vi "ReadDataUV-visSD.vi"(0 "Nombre de aq":i32=2, 1 "Binning Horizontal":i32=1) -> (2 "Channel I":i32[][](array[numeric]), 3 "Channel II":i32[][](array[numeric]), 4 "DLL error code":u32=20066, 5 "temps d'acqu ms":u32=4148)   [LabVIEW 2015]
uses:
  Error Code Enum typedef.ctl
panel:
  out "status":T1=enum."DRV_IDLE"
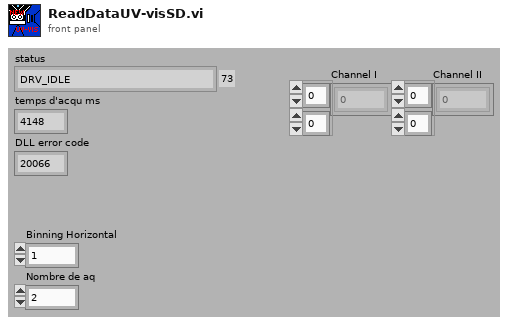
[diagram p1: front panel]
types:
  T1 = typedef "Error Code Enum typedef.ctl" = enum32{"N/A (0)", "DRV_ERROR_CODES", "DRV_SUCCESS", "DRV_VXDNOTINSTALLED", "DRV_ERROR_SCAN", "DRV_ERROR_CHECK_SUM", "DRV_ERROR_FILELOAD", "DRV_UNKNOWN_FUNC", "DRV_ERROR_VXD_INIT", "DRV_ERROR_ADDRESS", "DRV_ERROR_PAGELOCK", "DRV_ERROR_PAGEUNLOCK", "DRV_ERROR_BOARDTEST", "DRV_ERROR_ACK", "DRV_ERROR_UP_FIFO", "DRV_ERROR_PATTERN", "N/A (16)", "DRV_ACQUISITION_ERRORS", "DRV_ACQ_BUFFER", "DRV_ACQ_DOWNFIFO_FULL", "DRV_PROC_UNKONWN_INSTRUCTION", "DRV_ILLEGAL_OP_CODE", "DRV_KINETIC_TIME_NOT_MET", "DRV_ACCUM_TIME_NOT_MET", "DRV_NO_NEW_DATA", "N/A (25)", "DRV_SPOOLERROR", "N/A (27)", "N/A (28)", "N/A (29)", "N/A (30)", "N/A (31)", "N/A (32)", "DRV_TEMPERATURE_CODES", "DRV_TEMPERATURE_OFF", "DRV_TEMPERATURE_NOT_STABILIZED", "DRV_TEMPERATURE_STABILIZED", "DRV_TEMPERATURE_NOT_REACHED", "DRV_TEMPERATURE_OUT_RANGE", "DRV_TEMPERATURE_NOT_SUPPORTED", "DRV_TEMPERATURE_DRIFT", "N/A (41)", "N/A (42)", "N/A (43)", "N/A (44)", "N/A (45)", "N/A (46)", "N/A (47)", "N/A (48)", "DRV_GENERAL_ERRORS", "DRV_INVALID_AUX", "DRV_COF_NOTLOADED", "DRV_FPGAPROG", "DRV_FLEXERROR", "DRV_GPIBERROR", "N/A (55)", "N/A (56)", "N/A (57)", "N/A (58)", "N/A (59)", "N/A (60)", "N/A (61)", "N/A (62)", "N/A (63)", "DRV_DATATYPE", "DRV_DRIVER_ERRORS", "DRV_P1INVALID", "DRV_P2INVALID", "DRV_P3INVALID", "DRV_P4INVALID", "DRV_INIERROR", "DRV_COFERROR", "DRV_ACQUIRING", "DRV_IDLE", "DRV_TEMPCYCLE", "DRV_NOT_INITIALIZED", "DRV_P5INVALID", "DRV_P6INVALID", "DRV_INVALID_MODE", "DRV_INVALID_FILTER", "DRV_I2CERRORS", "DRV_I2CDEVNOTFOUND", "DRV_I2CTIMEOUT", "DRV_P7INVALID", "N/A (84)", "N/A (85)", "N/A (86)", "N/A (87)", "N/A (88)", "N/A (89)", "DRV_IOCERROR", "DRV_VRMVERSIONERROR"}
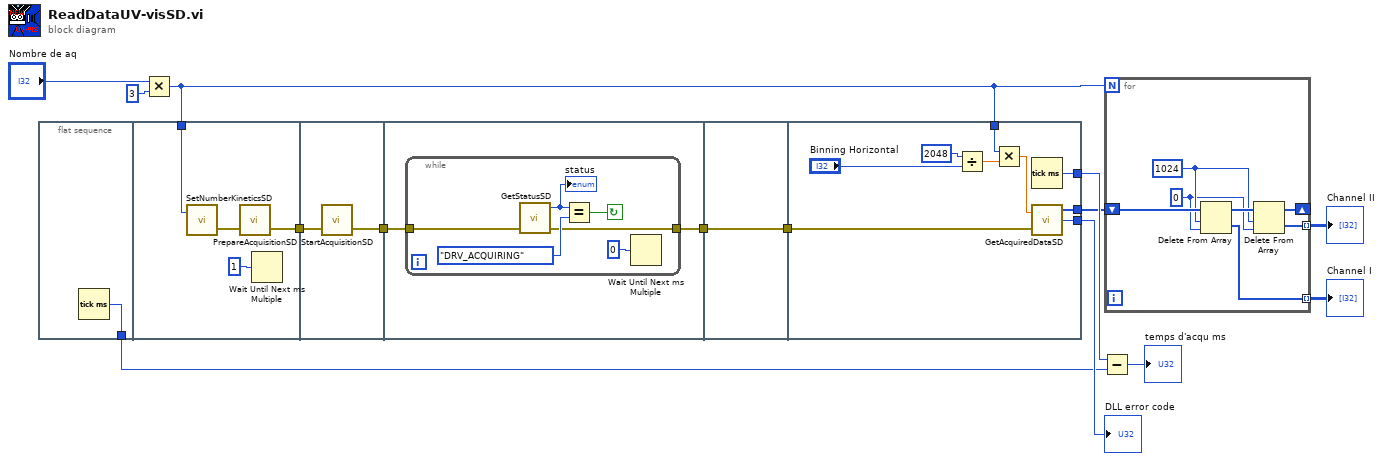
[diagram p0: block diagram]
diagram:
  n1 = flat-sequence {
    tunnel: [w15] -> w8
    tunnel: [w17] -> w12
    tunnel: w4 -> [w16]
    tunnel: w12 -> [w21]
    tunnel: [w20] -> w11
    tunnel: w11 -> [w23]
    tunnel: [w22] -> w9
    tunnel: [w30] -> w10
    tunnel: w9 -> [w30]
    tunnel: [w38] -> w3
    tunnel: [w37] -> w14
    tunnel: w10 -> [w34]
    tunnel: [w33] -> w7
    tunnel: w4 -> [w32]
    frame #0 {
      n2 = Tick Count (ms)() -> (millisecond timer value=w15:u32)
    }
    frame #1 {
      n3 = call "SetNumberKineticsSD.vi"("number"=w16) -> ("error out"=w19:errorcluster)  [unwired: 1 in, 1 out]
      n4 = call "PrepareAcquisitionSD.vi"("error in (no error)"=w19) -> ("error out"=w17:errorcluster)  [unwired: 1 in, 1 out]
      n5 = Wait Until Next ms Multiple(millisecond multiple=u32 1 ("n millisecondes")) -> ()  [unwired: 1 out]
    }
    frame #2 {
      n6 = call "StartAcquisitionSD.vi"("error in (no error)"=w21) -> ("error out"=w20:errorcluster)  [unwired: 1 in, 1 out]
    }
    frame #3 {
      n7 = while {
        tunnel: w23 -> [w25]
        tunnel: [w24] -> w22
        stop <- w27 continue-if-true
        n8 = call "GetStatusSD.vi"("error in (no error)"=w25) -> ("error out"=w24:errorcluster, "status"=w26:T1)  [unwired: 2 in, 1 out]
        "status" <- w26
        n9 = Equal?(x=w26, y=Error_Code_Enum_typedef."DRV_ACQUIRING") -> (x = y?=w27:bool)
        n10 = Wait Until Next ms Multiple(millisecond multiple=u32 0 ("n millisecondes")) -> ()  [unwired: 1 out]
      }
    }
    frame #4 {
    }
    frame #5 {
      n11 = Divide(x=2048 ("y"), y="Binning Horizontal") -> (x/y=w36:dbl)
      n12 = Multiply(x=w32, y=w36) -> (x*y=w39:dbl)
      n13 = Tick Count (ms)() -> (millisecond timer value=w33:u32)
      n14 = call "GetAcquiredDataSD.vi"("size"=w39, "error in (no error)"=w34) -> ("array"=w38:i32[], "DLL error code"=w37:u32)  [unwired: 1 out]
    }
  }
  n15 = Multiply(x="Nombre de aq", y=3) -> (x*y=w4:i32)
  n16 = Subtract(x=w7, y=w8) -> (x-y=→"temps d'acqu ms":u32)
  n17 = for {
    N: w4 -> [_]
    shift-right: [w40] -> _
    shift-left: w3 -> [w46]
    tunnel: [w45] -> w2 mode=indexing
    tunnel: [w41] -> w1 mode=indexing
    w42 = 0 ("index")
    w43 = 1024 ("length")
    n18 = Delete From Array(array=w46, length=w43, index=w42) -> (deleted portion=w45:i32[], array with subset deleted=w44:i32[])
    n19 = Delete From Array(array=w44, length=w43, index=w42) -> (deleted portion=w41:i32[], array with subset deleted=w40:i32[])
  }
  "Channel I" <- w2
  "Channel II" <- w1
  "DLL error code" <- w14
